vi "Write Message.vi"(8 "error in (no error)":errorcluster, 9 "Message Text":string, 10 "Message Name":T1, 11 "Sim Display Console Actor in":refnum<class "Sim Display Console Actor.lvclass">) -> (0 "error out":errorcluster, 3 "Sim Display Console Actor out":refnum<class "Sim Display Console Actor.lvclass">)   [LabVIEW 2019, in "Sim Display Console Actor.lvlib" / "Sim Display Console Actor.lvclass"]
uses:
  Sim Display Console Actor.lvclass
  Message Name.ctl
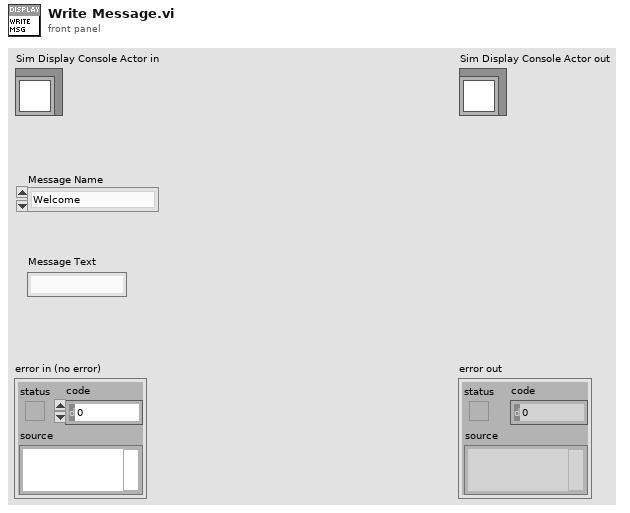
[diagram p1: front panel]
types:
  T1 = typedef "Sim Display Console Actor.lvlib/Sim Display Console Actor.lvclass/Message Name.ctl" = enum16{"Welcome", "Login", "Idle", "Invalid Login", "Terminate Session", "Deposit", "Withdrawal", "Fast Cash $50", "Withdrawal Complete", "Withdrawal Failed", "Balance Inquiry"}
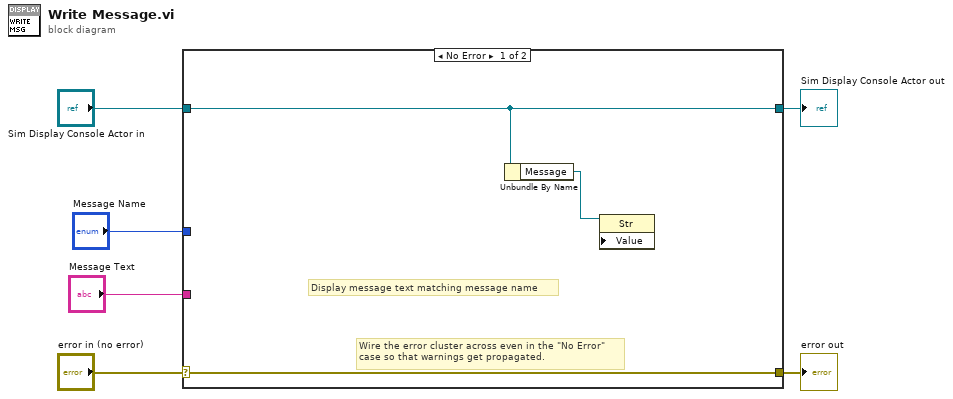
[diagram p0: block diagram]
diagram:
  n1 = case shown="No Error" "error in (no error)" {
    selector: "error in (no error)" -> [w9 w11]
    tunnel: [w9 w11] -> w5
    tunnel: [w7 w10] -> w3
    tunnel: "Sim Display Console Actor in" -> [w7 w10]
    tunnel: "Message Name" -> [_ _]
    tunnel: "Message Text" -> [_ _]
    frame No Error {
      # "Display message text matching message name"
      # "Wire the error cluster across even in the \"No Error\"\ncase so that warnings get propagated."
      n2 = Unbundle By Name(w7) -> ("Message"=w8:refnum<vi>)
      n3 = property class="Str" props=["Value"](reference=w8) -> ()  [unwired: 2 in, 2 out]
    }
    frame Error {
    }
  }
  "error out" <- w5
  "Sim Display Console Actor out" <- w3
